vi "l2n1.vi"() -> ()   [LabVIEW 2017]
panel:
  out "external indicator":dbl
  out "internal indicator":dbl
  in  "Numeric":dbl
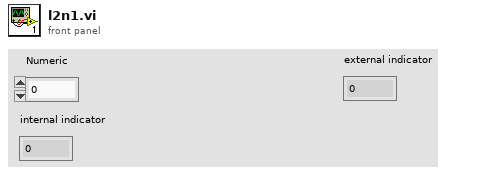
[diagram p1: front panel]
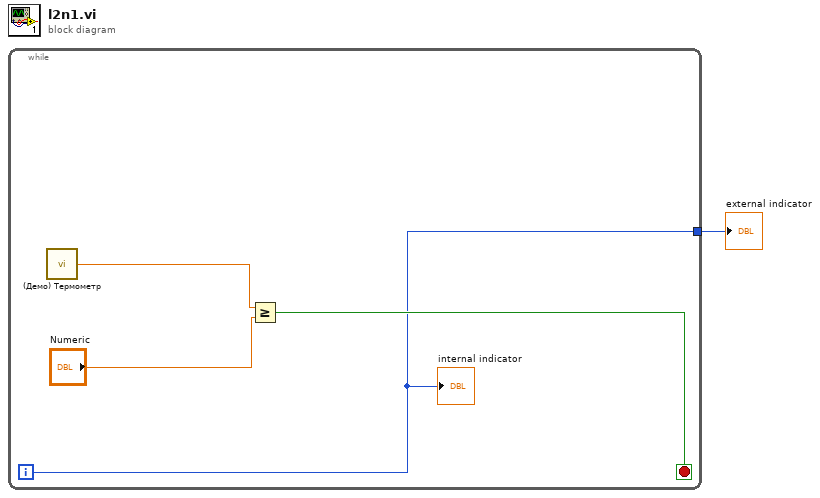
[diagram p0: block diagram]
diagram:
  n1 = while {
    tunnel: [w4] -> w1
    i -> [w4]
    stop <- w5 stop-if-true
    n2 = call "(Демо) Термометр.vi"() -> ("Температура"=w3:dbl)  [unwired: 1 in]
    n3 = Greater Or Equal?(x=w3, y="Numeric") -> (x >= y?=w5:bool)
    "internal indicator" <- w4
  }
  "external indicator" <- w1
